vi "Proiect IV.vi"() -> ()   [LabVIEW 2021]
uses:
  <vilib>/Instr/_visa.llb/VISA Configure Serial Port (Instr).vi
panel:
  in  "stop":bool
  in  "D13":bool
  in  "D9":bool
  in  "D5":bool
  in  "D12":bool
  in  "D8":bool
  in  "D4":bool
  in  "D11":bool
  in  "D7":bool
  in  "D3":bool
  in  "D10":bool
  in  "D6":bool
  in  "D2":bool
  in  "VISA resource name":refnum<visa-resource-name>
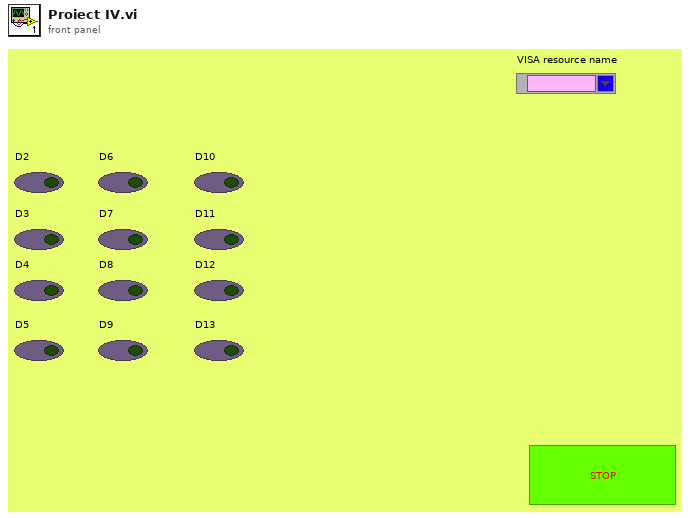
[diagram p1: front panel]
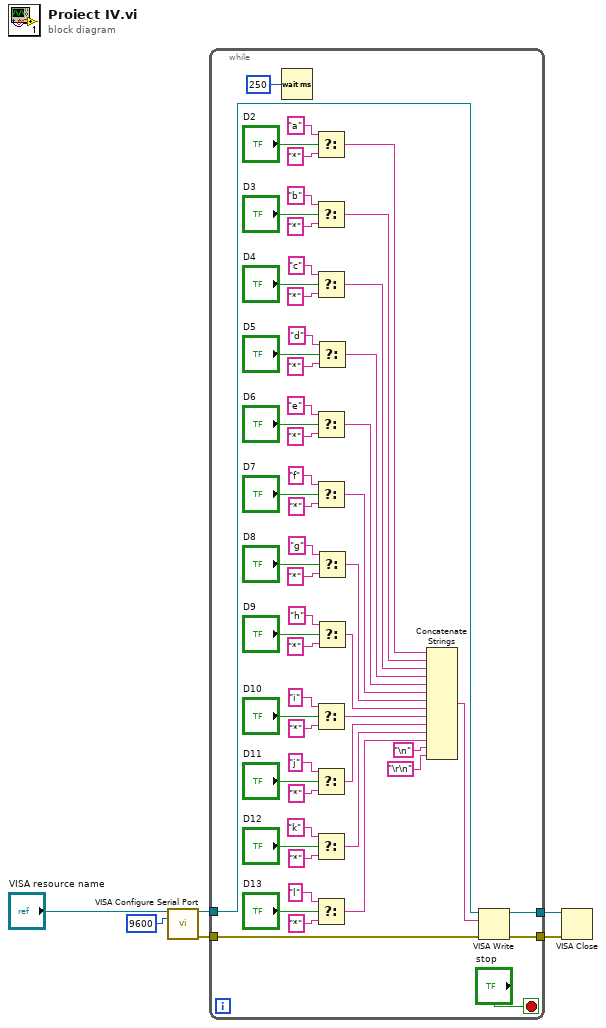
[diagram p0: block diagram]
diagram:
  n1 = call-poly "VISA Configure Serial Port"("VISA resource name"="VISA resource name", "baud rate (9600)"=u32 9600) -> ("VISA resource name out"=w4:refnum<visa-resource-name>, "error out"=w3:errorcluster)  [unwired: 12 in]
  n2 = while {
    tunnel: w4 -> [w15]
    tunnel: w3 -> [w16]
    tunnel: [w14] -> w2
    tunnel: [w13] -> w1
    stop <- "stop" stop-if-true
    n3 = Wait (ms)(milliseconds to wait=u32 250) -> ()  [unwired: 1 out]
    n4 = Select(t="a", s="D2", f="*") -> (s? t:f=w60:string)
    n5 = Select(t="b", s="D3", f="*") -> (s? t:f=w59:string)
    n6 = Select(t="c", s="D4", f="*") -> (s? t:f=w58:string)
    n7 = Select(t="e", s="D6", f="*") -> (s? t:f=w56:string)
    n8 = Select(t="f", s="D7", f="*") -> (s? t:f=w55:string)
    n9 = Select(t="i", s="D10", f="*") -> (s? t:f=w52:string)
    n10 = Select(t="j", s="D11", f="*") -> (s? t:f=w51:string)
    n11 = Select(t="k", s="D12", f="*") -> (s? t:f=w11:string)
    n12 = Select(t="l", s="D13", f="*") -> (s? t:f=w10:string)
    n13 = Select(t="d", s="D5", f="*") -> (s? t:f=w57:string)
    n14 = Select(t="g", s="D8", f="*") -> (s? t:f=w54:string)
    n15 = Select(t="h", s="D9", f="*") -> (s? t:f=w53:string)
    n16 = Concatenate Strings(w60, w59, w58, w57, w56, w55, w54, w53, w52, w51, w11, w10, "\n" ("Line Feed Constant"), "\r\n" ("End of Line Constant")) -> (w17:string)
    n17 = VISA Write(VISA resource name=w15, write buffer=w17, error in (no error)=w16) -> (VISA resource name out=w14:refnum<visa-resource-name>, error out=w13:errorcluster)  [unwired: 1 out]
  }
  n18 = VISA Close(VISA resource name=w2, error in (no error)=w1) -> ()  [unwired: 1 out]
